vi "MDPtr TotalCounter.vi"(6 "Oper(Get)":enum16{"GET", "Increament", "decreament"}(ring), 8 "error in (no error)":errorcluster) -> (0 "error out":errorcluster, 2 "Value out":i64)   [LabVIEW 2017, in "MDPtr.lvlib"]
uses:
  MDPtr.lvlib
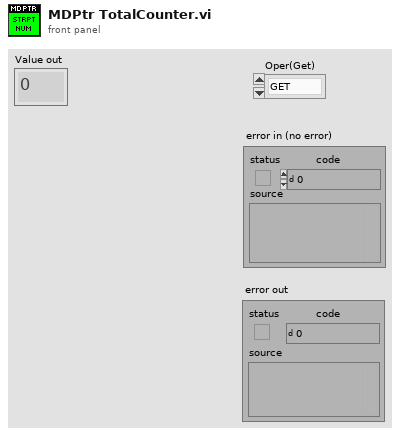
[diagram p1: front panel]
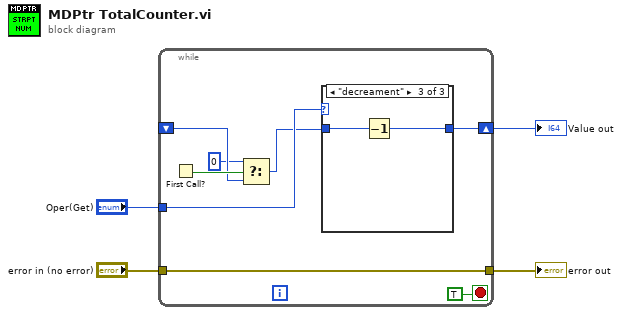
[diagram p0: block diagram]
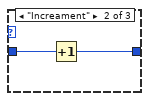
[diagram p3: hidden frame]
diagram:
  n1 = while {
    tunnel: "Oper(Get)" -> [w11]
    shift-right: [w10] -> w3
    shift-left: _ -> [w7]
    tunnel: "error in (no error)" -> [w9]
    tunnel: [w9] -> w1
    stop <- TRUE stop-if-true
    n2 = First Call?() -> (First Call?: T/F=w8:bool)
    n3 = Select(t=i64 0 ("Value in"), s=w8, f=w7) -> (s? t:f=w6:i64)
    n4 = case shown="\"decreament\"" w11 {
      tunnel: [w13 w14 w16] -> w10
      tunnel: w6 -> [w13 w15 w17]
      frame "GET", Default {
      }
      frame "Increament" {
        n5 = Increment(x=w15) -> (x+1=w14:i64)
      }
      frame "decreament" {
        n6 = Decrement(x=w17) -> (x-1=w16:i64)
      }
    }
  }
  "error out" <- w1
  "Value out" <- w3
